vi "Get_Pulse_Seq_DAQ.vi"(8 "error in":errorcluster, 11 "Filename (ini)":string="Config_Ver_2\\state_library") -> (0 "error out":errorcluster, 3 "data":T2)   [LabVIEW 2021]
uses:
  DAQ_Control_1.ctl
  DAQ_Control_2.ctl
  DAQ_Control_3 .ctl
  Global_DAQ.vi
  <vilib>/Utility/config.llb/NI_LVConfig.lvlib
panel:
  out "Time Unit":T1(ring)
  out "Sample  Frequency (Hz)":u32
  out "Sample Numbers":u32
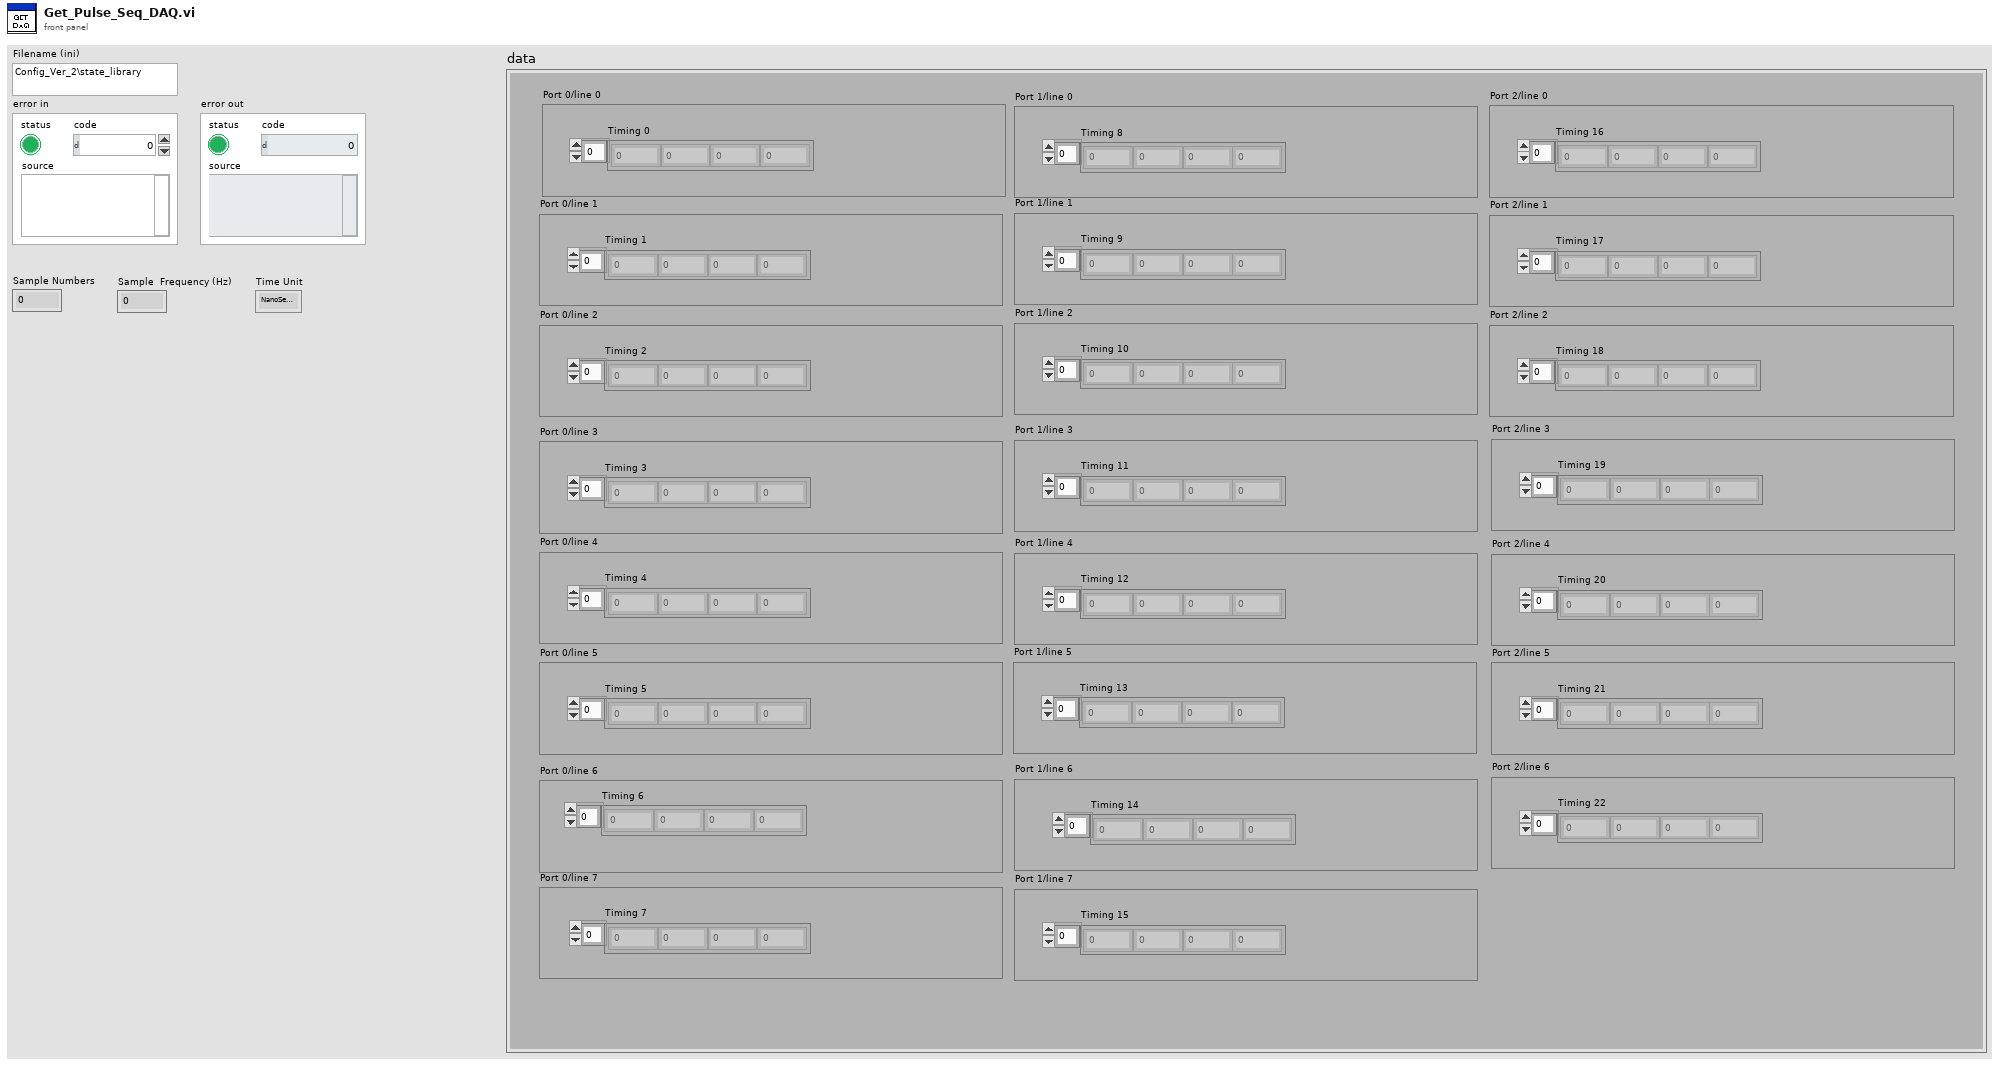
[diagram p1: front panel]
types:
  T1 = enum16{"NanoSecond", "MicroSecond", "MilliSecond"}
  T2 = typedef "DAQ_Control_1.ctl" = cluster{"Port 2/line 6":cluster{"Timing 22":dbl[]}, "Port 2/line 5":cluster{"Timing 21":dbl[]}, "Port 2/line 4":cluster{"Timing 20":dbl[]}, "Port 2/line 3":cluster{"Timing 19":dbl[]}, "Port 2/line 2":cluster{"Timing 18":dbl[]}, "Port 2/line 1":cluster{"Timing 17":dbl[]}, "Port 2/line 0":cluster{"Timing 16":dbl[]}, "Port 1/line 7":cluster{"Timing 15":dbl[]}, "Port 1/line 6":cluster{"Timing 14":dbl[]}, "Port 1/line 5":cluster{"Timing 13":dbl[]}, "Port 1/line 4":cluster{"Timing 12":dbl[]}, "Port 1/line 3":cluster{"Timing 11":dbl[]}, "Port 1/line 2":cluster{"Timing 10":dbl[]}, "Port 1/line 1":cluster{"Timing 9":dbl[]}, "Port 1/line 0":cluster{"Timing 8":dbl[]}, "Port 0/line 7":cluster{"Timing 7\n":dbl[]}, "Port 0/line 6":cluster{"Timing 6\n":dbl[]}, "Port 0/line 5":cluster{"Timing 5\n":dbl[]}, "Port 0/line 4":cluster{"Timing 4\n":dbl[]}, "Port 0/line 3":cluster{"Timing 3\n":dbl[]}, "Port 0/line 2":cluster{"Timing 2":dbl[]}, "Port 0/line 1":cluster{"Timing 1\n":dbl[]}, "Port 0/line 0":cluster{"Timing 0":dbl[]}}
  T3 = typedef "DAQ_Control_3 .ctl" = cluster{"Time Unit":enum16{"NanoSecond", "MicroSecond", "MilliSecond"}}
  T4 = typedef "DAQ_Control_2.ctl" = cluster{"Sample Numbers":u32, "Sample  Frequency (Hz)":u32}
  T5 = typedef "NI_LVConfig.lvlib/Config Data RefNum.ctl" = refnum<k1>
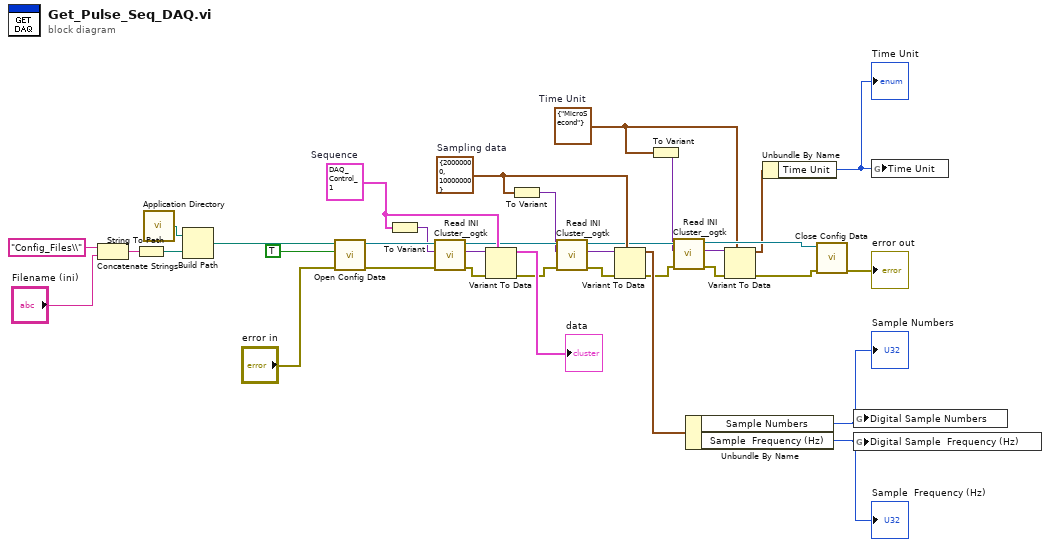
[diagram p0: block diagram]
diagram:
  w2 = T3 {"Time Unit"=enum."MicroSecond"}  # Time Unit
  w19 = T4 {"Sample Numbers"=20000000, "Sample  Frequency (Hz)"=10000000}  # Sampling data
  w22 = T2 {"Port 2/line 6"={"Timing 22"=[]}, "Port 2/line 5"={"Timing 21"=[]}, "Port 2/line 4"={"Timing 20"=[]}, "Port 2/line 3"={"Timing 19"=[]}, "Port 2/line 2"={"Timing 18"=[]}, "Port 2/line 1"={"Timing 17"=[]}, "Port 2/line 0"={"Timing 16"=[]}, "Port 1/line 7"={"Timing 15"=[]}, "Port 1/line 6"={"Timing 14"=[]}, "Port 1/line 5"={"Timing 13"=[]}, "Port 1/line 4"={"Timing 12"=[]}, "Port 1/line 3"={"Timing 11"=[]}, "Port 1/line 2"={"Timing 10"=[]}, "Port 1/line 1"={"Timing 9"=[]}, "Port 1/line 0"={"Timing 8"=[]}, "Port 0/line 7"={"Timing 7\n"=[]}, "Port 0/line 6"={"Timing 6\n"=[]}, "Port 0/line 5"={"Timing 5\n"=[]}, "Port 0/line 4"={"Timing 4\n"=[]}, "Port 0/line 3"={"Timing 3\n"=[]}, "Port 0/line 2"={"Timing 2"=[]}, "Port 0/line 1"={"Timing 1\n"=[]}, "Port 0/line 0"={"Timing 0"=[]}}  # Sequence
  n1 = Concatenate Strings("Config_Files\\" ("string"), "Filename (ini)") -> (w31:string)
  n2 = String To Path(string=w31) -> (path=w33:path)
  n3 = call <vilib>:"Application Directory.vi"() -> ("Application Directory"=w35:path)
  n4 = Build Path(base path=w35, name or relative path=w33) -> (appended path=w30:path)
  n5 = call <vilib>:"Open Config Data.vi"("error in (no error)"="error in", "create file if necessary (T)"=TRUE, "configuration file path"=w30) -> ("error out"=w26:errorcluster, "refnum"=w27:T5)  [unwired: 6 in, 1 out]
  n6 = To Variant(anything=w22) -> (Variant=w23:variant)
  n7 = call <userlib>:"Read INI Cluster__ogtk.vi"("error in (no error)"=w26, "INI Fomatted Cluster Type"=w23, "refnum"=w27) -> ("error out"=w16:errorcluster, "INI Fomatted Cluster"=w25:variant, "dup refnum"=w21:T5)  [unwired: 4 in, 2 out]
  n8 = Variant To Data(error in=w16, type=w22, Variant=w25) -> (data=→"data":T2, error out=w15:errorcluster)
  n9 = To Variant(anything=w19) -> (Variant=w20:variant)
  n10 = call <userlib>:"Read INI Cluster__ogtk.vi"("error in (no error)"=w15, "INI Fomatted Cluster Type"=w20, "refnum"=w21) -> ("error out"=w14:errorcluster, "INI Fomatted Cluster"=w18:variant, "dup refnum"=w10:T5)  [unwired: 4 in, 2 out]
  n11 = Variant To Data(error in=w14, type=w19, Variant=w18) -> (data=w17:T4, error out=w9:errorcluster)
  n12 = To Variant(anything=w2) -> (Variant=w4:variant)
  n13 = call <userlib>:"Read INI Cluster__ogtk.vi"("error in (no error)"=w9, "INI Fomatted Cluster Type"=w4, "refnum"=w10) -> ("error out"=w8:errorcluster, "INI Fomatted Cluster"=w5:variant, "dup refnum"=w6:T5)  [unwired: 4 in, 2 out]
  n14 = Unbundle By Name(w17) -> ("Sample Numbers"=w11:u32, "Sample  Frequency (Hz)"=w12:u32)
  "Sample Numbers" <- w11
  "Sample  Frequency (Hz)" <- w12
  n15 = Variant To Data(error in=w8, type=w2, Variant=w5) -> (data=w3:T3, error out=w7:errorcluster)
  n16 = Unbundle By Name(w3) -> ("Time Unit"=w1:T1)
  "Time Unit" <- w1
  n17 = call <vilib>:"Close Config Data.vi"("error in (no error)"=w7, "refnum"=w6) -> ("error out"=→"error out":errorcluster)  [unwired: 8 in, 1 out]
  n18 = global write "Global_DAQ.vi" "Digital Sample Numbers"(w11) -> ()
  n19 = global write "Global_DAQ.vi" "Digital Sample  Frequency (Hz)"(w12) -> ()
  n20 = global write "Global_DAQ.vi" "Time Unit"(w1) -> ()
